vi "Abort.vi"(8 "error in (no error)":errorcluster, 11 "Parallell Test Runner in":refnum<class "Parallell Test Runner.lvclass">) -> (0 "error out":errorcluster)   [LabVIEW 2020, in "Parallell Test Runner.lvclass"]
uses:
  Parallell Test Runner.lvclass
  Parallell Test Runner.lvclass/Parallell Test Runner.ctl
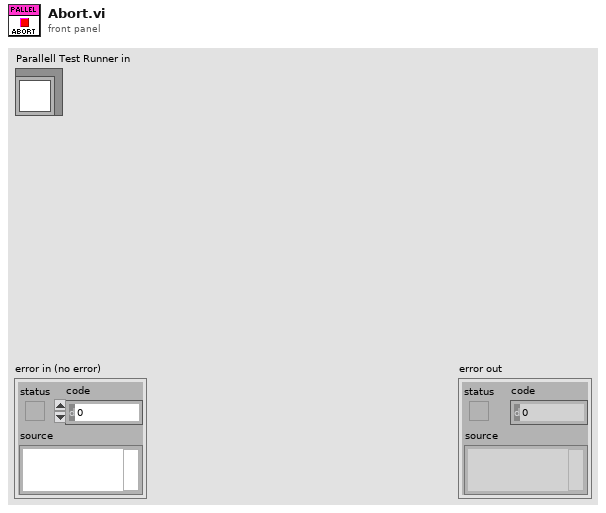
[diagram p1: front panel]
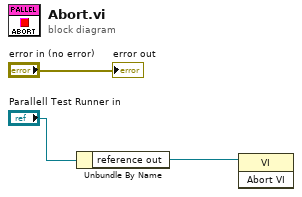
[diagram p0: block diagram]
diagram:
  n1 = Unbundle By Name("Parallell Test Runner in") -> ("reference out"=w1:refnum<vi>)
  n2 = invoke class="VI" method="Abort VI"(reference=w1) -> ()  [unwired: 2 in, 3 out]
  "error out" <- "error in (no error)"
